vi "Robot Global Data.vi"() -> ()   [LabVIEW 2014]
doc: "This global VI can contain as many global variables as you need. Place a control on the panel, give it a good name. To read or write to it from a VI, drag the icon to the diagram of that VI. You can also drag from the project. Click on the node to change which global you access. You shouldn't have multiple locations writing to a global or it will cause a race-condition."
uses:
  <vilib>/Rock Robotics/WPI/Camera/WPI_CameraImageSize.ctl
  <vilib>/Rock Robotics/WPI/DriverStation/WPI_DriverStationRobotMode2.ctl
  Common Code/IMU Data.ctl
  Drivetrain Code/Drivetrain Control.ctl
  Drivetrain Code/Drivetrain Mode.ctl
  Common Code/Solenoid Command.ctl
panel:
  in  "Solenoid Command":T1
  in  "Drivetrain Command":T2={"Mode"=enum."Gyro Steer", "X"=0.0, "Y"=0.0, "Heading Target"=0.0, "Y Target"=0.0}
  in  "IMU Gyro Zero Z":dbl
  in  "IMU Gyro Zero Y":dbl
  in  "IMU Gyro Zero X":dbl
  out "IMU Data":T4
  in  "Robot Mode":T5
  in  "image size":T6=enum."320x240"
  in  "Enable Vision":bool
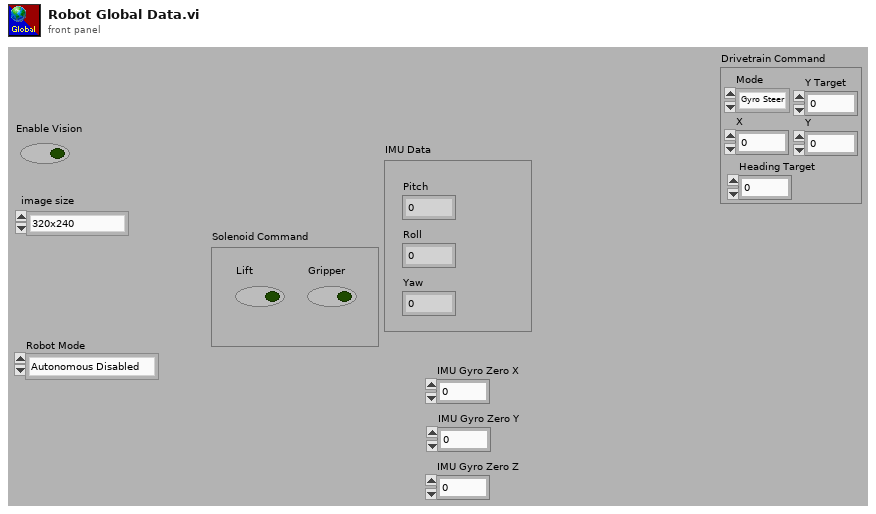
[diagram p1: front panel]
types:
  T1 = typedef "Solenoid Command.ctl" = cluster{"Lift":bool, "Gripper":bool}
  T2 = typedef "Drivetrain Control.ctl" = cluster{"Mode":T3, "X":dbl, "Y":dbl, "Heading Target":dbl, "Y Target":dbl}
  T3 = typedef "Drivetrain Mode.ctl" = enum16{"Manual", "Gyro Steer", "Vision Steer", "Drive Distance"}
  T4 = typedef "IMU Data.ctl" = cluster{"Pitch":sgl, "Roll":sgl, "Yaw":sgl}
  T5 = typedef "WPI_DriverStationRobotMode2.ctl" = enum16{"Autonomous Disabled", "Autonomous Enabled", "Teleop Disabled", "Teleop Enabled", "Disconnected", "Finish", "Test Disabled", "Test Enabled", "Emergency Stopped"}
  T6 = typedef "WPI_CameraImageSize.ctl" = enum16{"640x480", "320x240", "160x120", "Custom"}
diagram:
